vi "DrawSprites.vi"(8 "error in (no error)":errorcluster, 10 "Sprites in":refnum<class "RT_Sprite.lvclass">[](array[class]), 11 "Game in":refnum<class "Game.lvclass">) -> (0 "error out":errorcluster, 2 "Sprites out":refnum<class "RT_Sprite.lvclass">[](array[class]), 3 "Game out":refnum<class "Game.lvclass">)   [LabVIEW 2019, in "RT_Game.lvlib" / "Game.lvclass"]
uses:
  Game.lvclass
  RT_Sprite/RT_Sprite.lvclass
  C:/Users/FreshBob/Dropbox/VIs/myRIO_GameConsole/RT/RT_Game/GameObject/GameObject.lvclass
  Game.lvclass/Game.ctl
  FPGA/Sprite/SpriteData.ctl
  GameObject/GameObject.lvclass/GameObject.ctl
  RT_Sprite/RT_Sprite.lvclass/RT_Sprite.ctl
  GameObject/Read position.vi
  GameObject/Read size.vi
  GameObject/Read IsActive.vi
  RT_Sprite/Read TransparentColor.vi
  Read FPGA_ref.vi
  Write FPGA_ref.vi
  <vilib>/Utility/error.llb/Error Cluster From Error Code.vi
  <vilib>/rvi/errors/niLvFpgaAdjustHostInterfaceError.vi
  FPGA_Interface.ctl
  <vilib>/rvi/interface/nirviReadWriteControl/nirviReadWriteControl.xnode
  FPGA Bitfiles/myriogameconsole_FPGATarget_Main_ntsPRcBZGxk.lvbitx
  FPGA/Sprite/Sprite.lvlib
  NiFpgaLv.dll
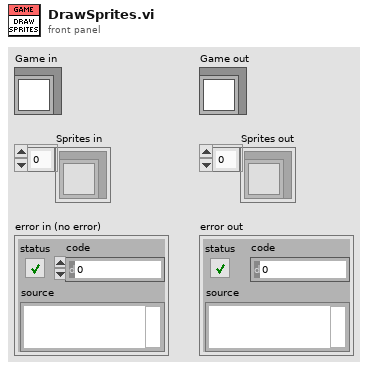
[diagram p1: front panel]
types:
  T1 = typedef "Sprite.lvlib/SpriteData.ctl" = cluster{"Pos_X":i16, "Pos_Y":i16, "Width":i16, "Height":i16, "BufferIndex":i16, "TransparencyColor":fxp<+,3,3>}
  T2 = typedef "RT_Game.lvlib/Game.lvclass/Coordinate.ctl" = cluster{"x":dbl, "y":dbl}
  T3 = typedef "FPGA_Interface.ctl" = refnum<k20>
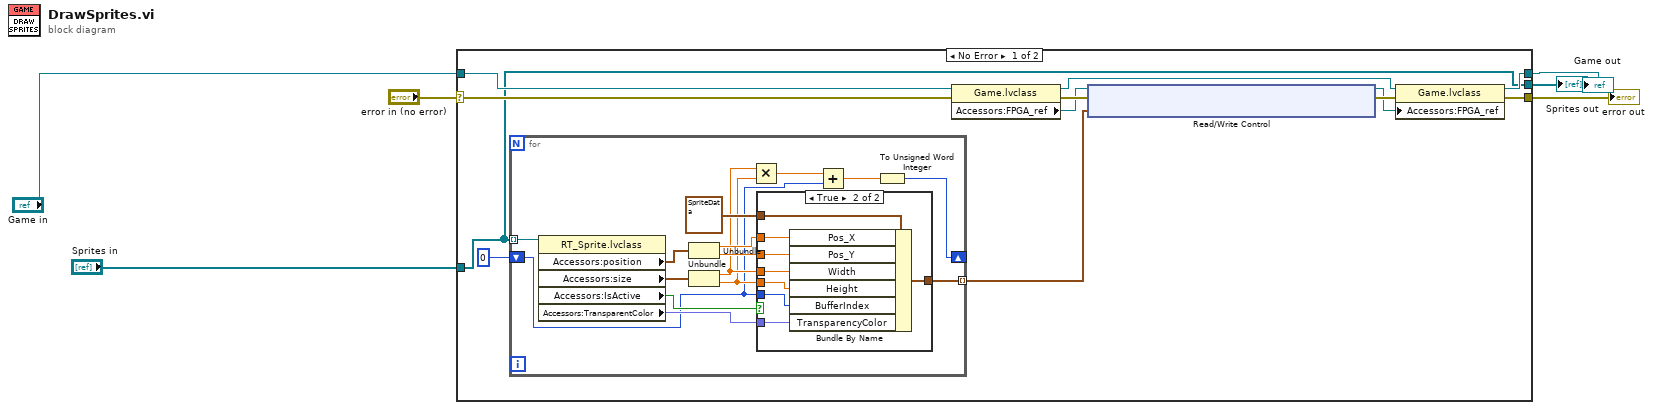
[diagram p0: block diagram]
diagram:
  n1 = case shown="No Error" "error in (no error)" {
    selector: "error in (no error)" -> [w13 w45]
    tunnel: [w14 w45] -> w2
    tunnel: [w8 w44] -> w4
    tunnel: "Sprites in" -> [w8 w44]
    tunnel: [w17 w43] -> w6
    tunnel: "Game in" -> [w18 w43]
    frame No Error {
      n2 = for {
        tunnel: [w31] -> w9 mode=indexing
        tunnel: w8 -> [w32] mode=indexing
        shift-right: [w19] -> _
        shift-left: u16 0 ("BufferIndex") -> [w20]
        n3 = property class="RT_Sprite.lvclass"(reference=w32) -> ("Accessors:position"=w30:T2, "Accessors:size"=w28:T2, "Accessors:IsActive"=w22:bool, "Accessors:TransparentColor"=w21:fxp<+,3,3>)  [unwired: 1 in, 2 out]
        n4 = Unbundle(w30) -> ("x"=w27:dbl, "y"=w29:dbl)
        n5 = Unbundle(w28) -> ("x"=w26:dbl, "y"=w25:dbl)
        n6 = Multiply(x=w26, y=w25) -> (x*y=w23:dbl)
        n7 = case shown="True" w22 {
          tunnel: T1 {"Pos_X"=0, "Pos_Y"=0, "Width"=0, "Height"=0, "BufferIndex"=0, "TransparencyColor"=0.0} ("Sprite1") -> [w34 w42]
          tunnel: [w34 w41] -> w31
          tunnel: w29 -> [_ w40]
          tunnel: w27 -> [_ w39]
          tunnel: w26 -> [_ w38]
          tunnel: w25 -> [_ w37]
          tunnel: w21 -> [_ w36]
          tunnel: w20 -> [_ w35]
          frame False {
          }
          frame True {
            n8 = Bundle By Name(cluster=w42, "Pos_X"=w39, "Pos_Y"=w40, "Width"=w38, "Height"=w37, "BufferIndex"=w35, "TransparencyColor"=w36) -> (w41:T1)
          }
        }
        n9 = Add(x=w23, y=w20) -> (x+y=w24:dbl)
        n10 = To Unsigned Word Integer(number=w24) -> (unsigned 16bit integer=w19:u16)
      }
      n11 = property class="Game.lvclass"(reference=w18, error in=w13) -> (reference out=w16:refnum<class "Game.lvclass">, error out=w15:errorcluster, "Accessors:FPGA_ref"=w11:T3)
      n12 = xnode "Read/Write Control"("FPGA VI Reference In"=w11, "error in"=w15, "Sprites"=w9) -> ("FPGA VI Reference Out"=w10:T3, "error out"=w12:errorcluster)
      n13 = property class="Game.lvclass"(reference=w16, error in=w12, "Accessors:FPGA_ref"=w10) -> (reference out=w17:refnum<class "Game.lvclass">, error out=w14:errorcluster)
    }
    frame Error {
    }
  }
  "Game out" <- w6
  "Sprites out" <- w4
  "error out" <- w2
